vi "Write ASCII Char.vi"(8 "error in (no error)":errorcluster, 9 "Char":string, 11 "LEDMatrix in":refnum<class "LEDMatrix.lvclass">) -> (0 "error out":errorcluster, 3 "LEDMatrix out":refnum<class "LEDMatrix.lvclass">)   [LabVIEW 2020, in "CTI-Peripheral.lvlib" / "LEDMatrix.lvclass"]
uses:
  LEDMatrix.lvclass
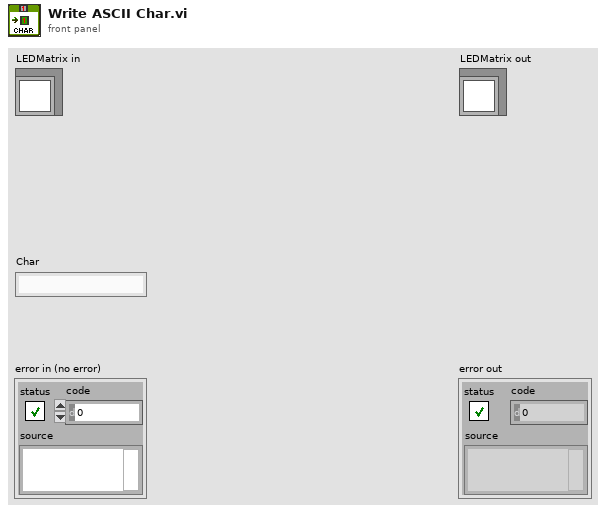
[diagram p1: front panel]
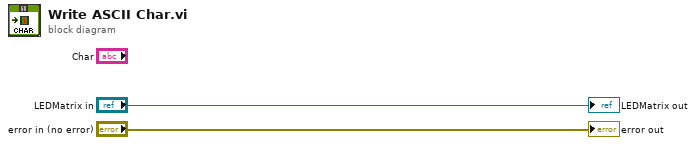
[diagram p0: block diagram]
diagram:
  "error out" <- "error in (no error)"
  "LEDMatrix out" <- "LEDMatrix in"
